vi "List Classes.vi"(8 "Error In":errorcluster, 11 "Class Path":path[](array[path])) -> (0 "Error Out":errorcluster, 2 "Class Names":string[](array[string]), 3 "DVR Ref":T1[](array[typedef]))   [LabVIEW 2019, in "Arithemetic Operation.lvclass"]
doc: "This method gets the array of paths of classes and separates the name of the classes and creates a DVR for each of the classes."
uses:
  Arithemetic Operation.lvclass
  Typedef/DVR Ref.ctl
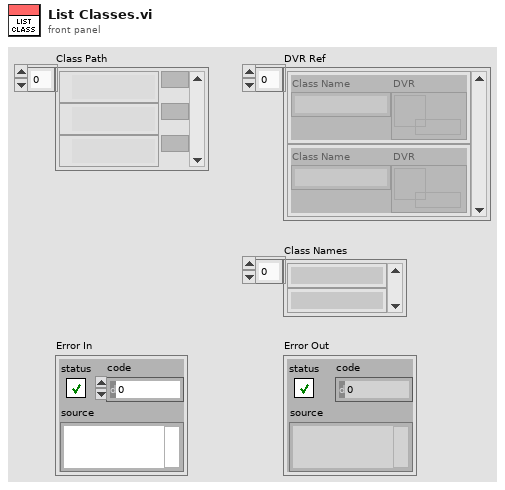
[diagram p1: front panel]
types:
  T1 = typedef "DVR Ref.ctl" = cluster{"Class Name":string, "DVR":refnum<data-value>}
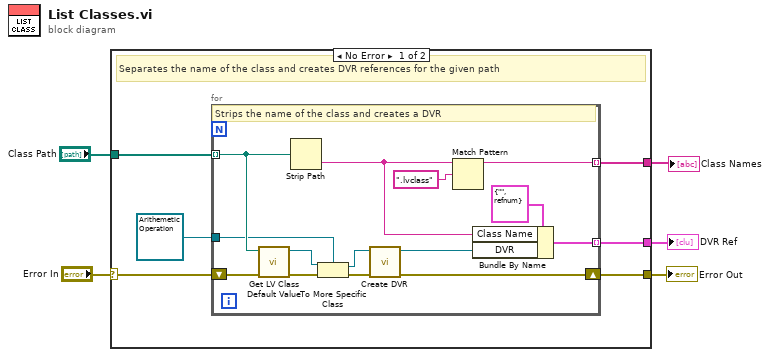
[diagram p0: block diagram]
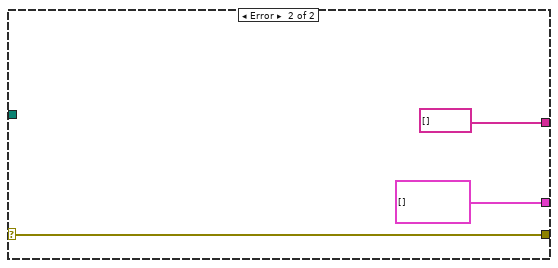
[diagram p2: hidden frame]
diagram:
  n1 = case shown="No Error" "Error In" {
    selector: "Error In" -> [w9 w28]
    tunnel: [w10 w28] -> w4
    tunnel: "Class Path" -> [w8 _]
    tunnel: [w7 T1[] []] -> w2
    tunnel: [w6 string[] []] -> w1
    frame No Error {
      # "Separates the name of the class and creates DVR references for the given path"
      n2 = for {
        tunnel: w8 -> [w22] mode=indexing
        tunnel: [w21] -> w6 mode=indexing
        shift-right: [w16] -> w10
        shift-left: w9 -> [w24]
        tunnel: refnum<class "Arithemetic Operation.lvclass"> refnum ("Arithemetic Operation in") -> [w19]
        tunnel: [w14] -> w7 mode=indexing
        # "Strips the name of the class and creates a DVR"
        n3 = call <vilib>:"Get LV Class Default Value.vi"("error in (no error)"=w24, "class path"=w22) -> ("error out"=w23:errorcluster, "object"=w18:refnum<class>)  [unwired: 8 in]
        n4 = Strip Path(path=w22) -> (name=w13:string)  [unwired: 1 out]
        n5 = To More Specific Class(target class=w19, reference=w18, error in=w23) -> (specific class reference=w15:refnum<class "Arithemetic Operation.lvclass">, error out=w20:errorcluster)
        n6 = call "Create DVR.vi"("Error In"=w20, "Arithmetic Class"=w15) -> ("Error Out"=w16:errorcluster, "DVR"=w12:refnum<data-value>)  [unwired: 8 in]
        n7 = Match Pattern(string=w13, regular expression=".lvclass") -> (before substring=w21:string)  [unwired: 1 in, 3 out]
        n8 = Bundle By Name(cluster=T1 {"Class Name"="", "DVR"=refnum}, "Class Name"=w13, "DVR"=w12) -> (w14:T1)
      }
    }
    frame Error {
    }
  }
  "Error Out" <- w4
  "DVR Ref" <- w2
  "Class Names" <- w1
